vi "amplitudeOscillation.vi"(1 "y0":dbl, 2 "x0":dbl, 3 "y2":dbl, 4 "x2":dbl, 5 "y1":dbl, 6 "x1":dbl) -> (0 "amplitudeOscillation":dbl)   [LabVIEW 2015]
panel:
  # "Si calcola considerando la differenza tra l'ampiezza del massimo meno la media delle ampiezze dei minimi relativi"
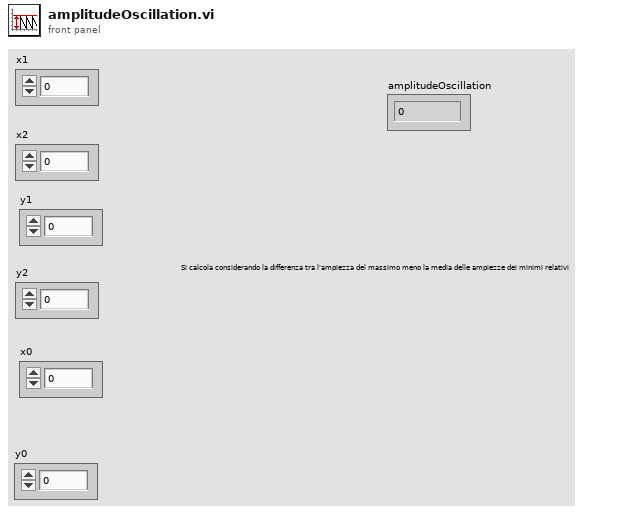
[diagram p1: front panel]
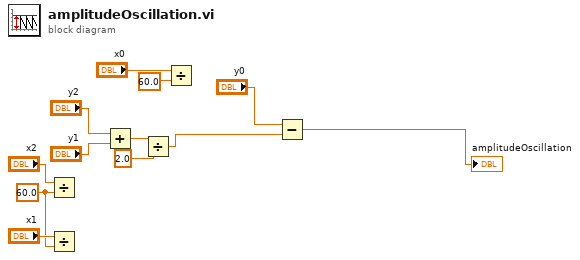
[diagram p0: block diagram]
diagram:
  w9 = 60.0 ("y")
  n1 = Divide(x="x2", y=w9) -> ()  [unwired: 1 out]
  n2 = Divide(x="x1", y=w9) -> ()  [unwired: 1 out]
  n3 = Add(x="y2", y="y1") -> (x+y=w5:dbl)
  n4 = Divide(x=w5, y=2.0) -> (x/y=w2:dbl)
  n5 = Divide(x="x0", y=60.0) -> ()  [unwired: 1 out]
  n6 = Subtract(x="y0", y=w2) -> (x-y=→"amplitudeOscillation":dbl)
